vi "Zan-WaitInId.vi"(6 "time(0.1)":i32=100, 8 "error in":errorcluster, 9 "Wait?":bool=TRUE, 10 "Status":bool, 11 "IO_Input":T1) -> (0 "error Out":errorcluster, 2 "TimeOut":bool, 3 "StatusOut":bool)   [LabVIEW 2015]
uses:
  Ctrl/Zan-64_SelectInPut.ctl
  Ctrl/IO Card_Type.ctl
  global/InAndOutGB.vi
  global/IO_FlagGB.vi
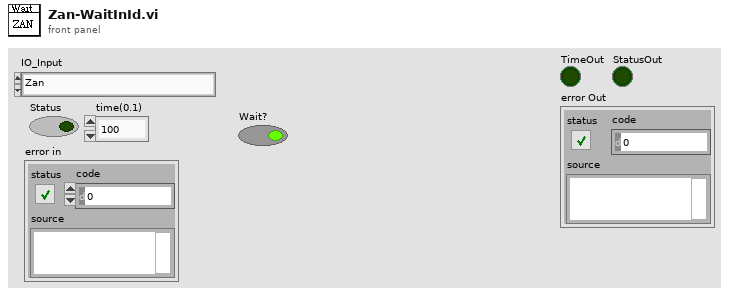
[diagram p1: front panel]
types:
  T1 = typedef "Zan-64_SelectInPut.ctl" = enum16{"Zan", "大料盤防呆檢知", "小料盤防呆檢知", "升降台有料檢知", "進料盤推到位檢知1", "進料盤推到位檢知2", "升降台檢速檢知", "升降台工作檢知", "大盤吸取汽缸上位", "大盤吸取汽缸下位", "小盤吸取汽缸上位", "小盤吸取汽缸下位", "大盤吸取真空檢知", "小盤吸取真空檢知1", "小盤吸取真空檢知2", "移載軸有盤檢知", "移載軸前位檢知 取料位", "移載軸後位檢知 放料位", "移載大盤靠位檢知 (開位)", "移載小盤靠位檢知 (開位)", "第一軸READY", "第二軸READY", "第三軸READY", "第四軸READY", "收料汽缸下位", "收料汽缸上位", "滿料檢知", "收料抽拉到位檢知", "第一軸INP", "第二軸INP", "第三軸INP", "第四軸INP"}
  T2 = typedef "IO Card_Type.ctl" = enum16{"None", "Unidaq32", "IPC_3005(9700)", "6480", "2410C-64", "Zan"}
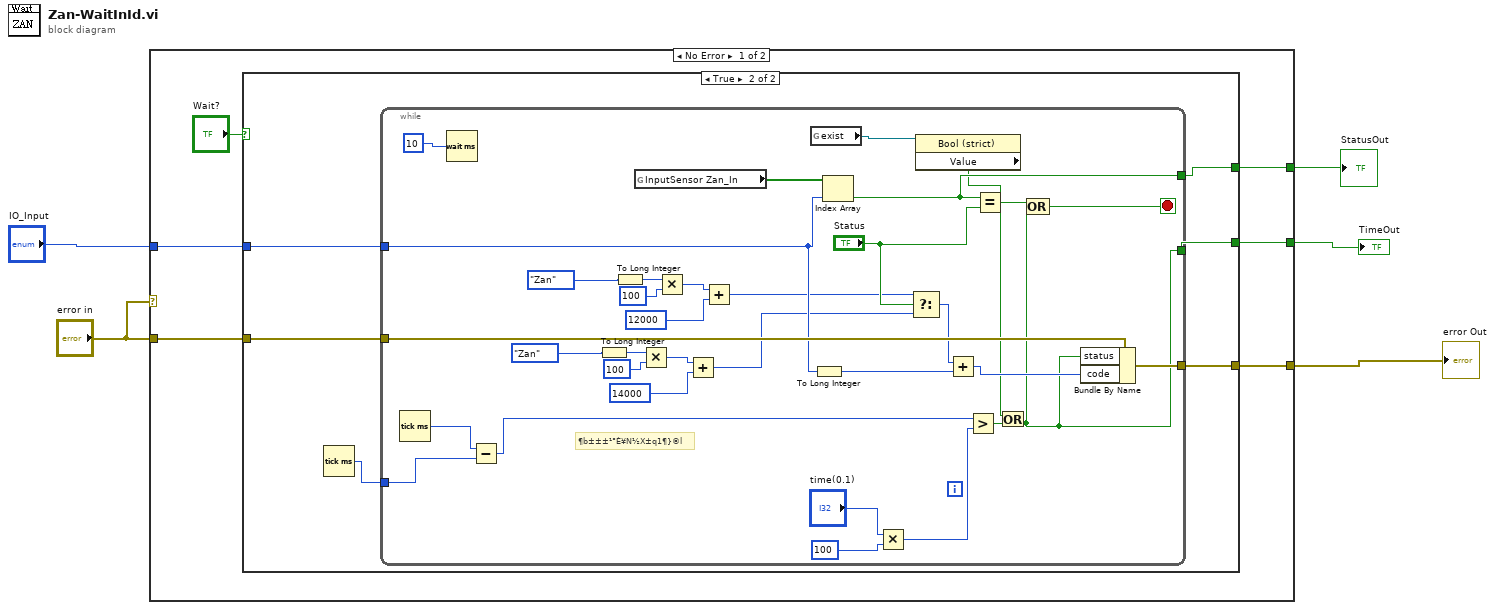
[diagram p0: block diagram]
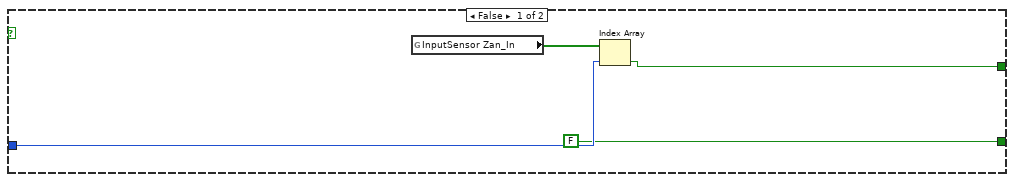
[diagram p2: hidden frame]
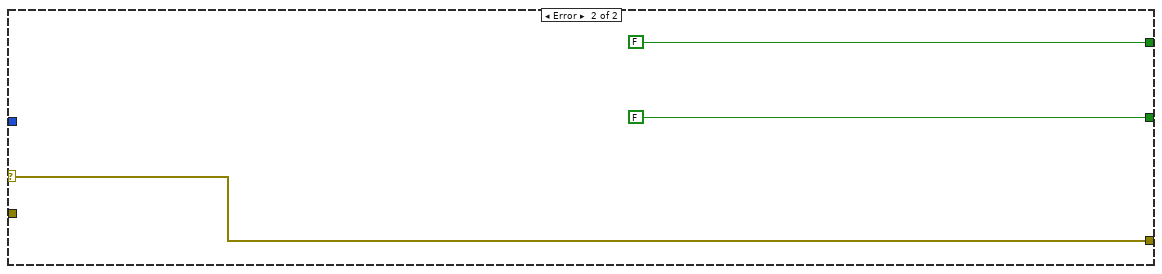
[diagram p3: hidden frame]
diagram:
  n1 = case shown="No Error" "error in" {
    selector: "error in" -> [_ w57]
    tunnel: [w11 FALSE] -> w5
    tunnel: "error in" -> [w10 _]
    tunnel: [w9 w57] -> w4
    tunnel: [w8 FALSE ("Boolean")] -> w2
    tunnel: "IO_Input" -> [w6 _]
    frame No Error {
      n2 = case shown="True" "Wait?" {
        tunnel: [FALSE w21] -> w11
        tunnel: w10 -> [_ w20]
        tunnel: [_ w19] -> w9
        tunnel: [w13 w18] -> w8
        tunnel: w6 -> [w14 w17]
        frame False {
          n3 = global read "InAndOutGB.vi" "InputSensor Zan_In"() -> (w15:bool[])
          n4 = Index Array(array=w15, index=w14) -> (element=w13:bool)
        }
        frame True {
          n5 = Tick Count (ms)() -> (millisecond timer value=w16:u32)
          n6 = while {
            tunnel: [w44] -> w21
            tunnel: w20 -> [w51]
            tunnel: [w48] -> w19
            tunnel: [w43] -> w18
            tunnel: w17 -> [w41]
            tunnel: w16 -> [w23]
            stop <- w53 stop-if-true
            # "¶b±±±¹°È¥N½X±q1¶}©l"
            n7 = Tick Count (ms)() -> (millisecond timer value=w24:u32)
            n8 = Wait (ms)(milliseconds to wait=u32 10) -> ()  [unwired: 1 out]
            n9 = Subtract(x=w24, y=w23) -> (x-y=w22:u32)
            n10 = To Long Integer(number=IO_Card_Type."Zan" ("IO Card Type")) -> (32bit integer=w30:i32)
            n11 = To Long Integer(number=IO_Card_Type."Zan" ("IO Card Type")) -> (32bit integer=w38:i32)
            n12 = global read "InAndOutGB.vi" "InputSensor Zan_In"() -> (w54:bool[])
            n13 = Multiply(x=w30, y=100) -> (x*y=w32:i32)
            n14 = Multiply(x=w38, y=100) -> (x*y=w36:i32)
            n15 = Add(x=w32, y=14000) -> (x+y=w28:i32)
            n16 = Add(x=w36, y=12000) -> (x+y=w34:i32)
            n17 = global read "IO_FlagGB.vi" "exist"() -> (w40:refnum<vi>)
            n18 = To Long Integer(number=w41) -> (32bit integer=w45:i32)
            n19 = Index Array(array=w54, index=w41) -> (element=w43:bool)
            n20 = Multiply(x="time(0.1)", y=u32 100 ("milliseconds to wait")) -> (x*y=w25:u32)
            n21 = Select(t=w34, s="Status", f=w28) -> (s? t:f=w46:i32)
            n22 = property class="Bool (strict)"(reference=w40) -> ("Value"=w42:bool)  [unwired: 1 in, 2 out]
            n23 = Add(x=w46, y=w45) -> (x+y=w49:i32)
            n24 = Greater?(x=w22, y=w25) -> (0:w50:bool)
            n25 = Equal?(x=w43, y="Status") -> (x = y?=w52:bool)
            n26 = Or(x=w42, y=w50) -> (x .or. y?=w44:bool)
            n27 = Compound Arithmetic op=OR(w52, w44) -> (w53:bool)
            n28 = Bundle By Name(cluster=w51, "status"=w44, "code"=w49) -> (w48:errorcluster)
          }
        }
      }
    }
    frame Error {
    }
  }
  "TimeOut" <- w5
  "error Out" <- w4
  "StatusOut" <- w2
